vi "PH_BL-Master.create DIM Services.vi"(0 "Refnum in":refnum<vi>, 2 "Create Services? (false)":bool, 5 "error in":errorcluster) -> (14 "i ref out":refnum<vi>, 19 "error out":errorcluster)   [LabVIEW 2014]
doc: "This VI creates DIM services."
uses:
  PH_BL-Master.lvlib
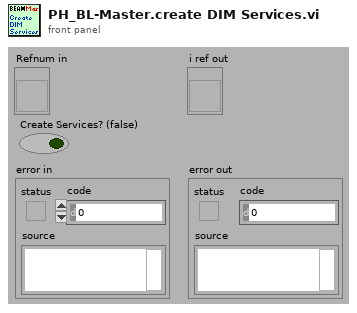
[diagram p1: front panel]
types:
  T1 = typedef "PH_BL-Master.lvlib/PH_BL-Master.i attribute.ctl" = cluster{"GUI Refs":cluster{"Delete":refnum<vi>}, "Remote Controlled by":string, "Boolean Condition Service Subscriber":refnum<vi>[], "Picture Condition Service Subscriber":refnum<vi>[], "R2S":cluster{"GUI Ref":refnum<vi>, "State":bool}, "Vacua":cluster{"GUI Ref":refnum<vi>, "Limit":dbl, "Curr Value":dbl, "in range":bool}[], "O2 Inspection":cluster{"GUI Ref":refnum<vi>, "Concentration":dbl, "State":T2}[], "Boolean Status Service Subscriber":cluster{"GUI Ref":refnum<vi>, "Status":T2, "no Link?":bool, "Status Subscriber Class":T3}[], "Picture Status Service Subscriber":cluster{"GUI Ref":refnum<vi>, "Status":T2, "no Link?":bool, "Status Subscriber Class":T3}[], "6P 4Q Service Subscriber":cluster{"GUI Ref":refnum<vi>, "Selector":T4, "no Link?":bool}[], "Index of latest 6P 4Q changing Instance":i32, "Index of latest Picture Status changing Instance":i32, "Index of latest Boolean Status changing Instance":i32, "Vision ID on same Node":string, "Start Phase over?":bool, "Chief?":bool}
  T2 = typedef "Status.ctl" = i16
  T3 = typedef "PH_BL-Master.lvlib/PH_BL-Master.Status Subscriber Class.ctl" = enum16{"unknown", "Switch", "BB", "6P Switch", "Switch GUI", "Switch and 6P State"}
  T4 = typedef "PH_4_Pos_Selector.lvlib/PH_4_Pos_Selector.Position Selector.ctl" = u16
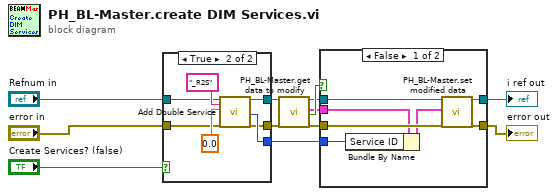
[diagram p0: block diagram]
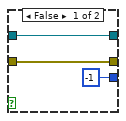
[diagram p2: hidden frame]
diagram:
  n1 = case shown="True" "Create Services? (false)" {
    tunnel: [w15 w22] -> w5
    tunnel: [-1 ("Service ID") w21] -> w6
    tunnel: [w14 w20] -> w7
    tunnel: "Refnum in" -> [w15 w17]
    tunnel: "error in" -> [w14 w16]
    frame False {
    }
    frame True {
      n2 = call "Add Double Service.vi"("i ref in"=w17, "Service Name"="_R2S" ("string"), "Double Value"=0.0 ("x"), "error in (no error)"=w16) -> ("i ref out"=w22:refnum<vi>, "Service ID"=w21:i32, "error out"=w20:errorcluster)  [unwired: 13 in]
    }
  }
  n3 = call "PH_BL-Master.get data to modify.vi"("i ref in"=w5, "error in (no error)"=w7) -> ("i ref out"=w1:refnum<vi>, "i attribute"=w3:T1, "timed out"=w4:bool, "error out"=w2:errorcluster)  [unwired: 14 in]
  n4 = case shown="False" w4 {
    tunnel: w1 -> [w29 w31]
    tunnel: [w28 w31] -> w10
    tunnel: w2 -> [w27 w30]
    tunnel: [w26 w30] -> w12
    tunnel: w3 -> [w25 _]
    tunnel: w6 -> [w23 _]
    frame False {
      n5 = Bundle By Name(cluster=w25, "Service ID"=w23) -> (w24:T1)
      n6 = call "PH_BL-Master.set modified data.vi"("i ref in"=w29, "i attribute"=w24, "error in (no error)"=w27) -> ("i ref out"=w28:refnum<vi>, "error out"=w26:errorcluster)  [unwired: 15 in]
    }
    frame True {
    }
  }
  "error out" <- w12
  "i ref out" <- w10
